vi "VI-Replace Event Type.vi"(7 "Event Data typedef":path, 11 "error in (no error)":errorcluster, 12 "Event Type typedef":path) -> (15 "error out":errorcluster)   [LabVIEW 2015]
uses:
  <vilib>/Utility/traverseref.llb/TRef TravTarget.ctl
  <vilib>/Utility/traverseref.llb/VI Scripting - Traverse.lvlib
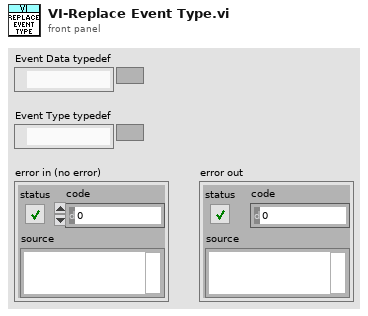
[diagram p1: front panel]
types:
  T1 = typedef "TRef TravTarget.ctl" = enum16{"FP", "BD", "Other"}
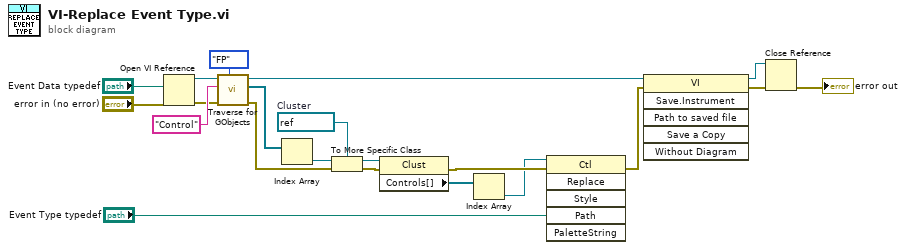
[diagram p0: block diagram]
diagram:
  w7 = refnum<vi> refnum  # Cluster
  n1 = Open VI Reference(vi path="Event Data typedef", error in (no error)="error in (no error)") -> (vi reference=w12:refnum<vi>, error out=w1:errorcluster)  [unwired: 4 in]
  n2 = call <vilib>:"Traverse for GObjects.vi"("Traverse Target"=TRef_TravTarget."FP", "error in (no error)"=w1, "Class Name"="Control", "VI Refnum"=w12) -> ("error out"=w4:errorcluster, "References"=w9:refnum<vi>[], "dup VI Refnum"=w16:refnum<vi>)  [unwired: 4 in, 1 out]
  n3 = Index Array(array=w9) -> (element=w8:refnum<vi>)  [unwired: 1 in]
  n4 = To More Specific Class(target class=w7, reference=w8, error in=w4) -> (specific class reference=w5:refnum<vi>, error out=w6:errorcluster)
  n5 = property class="Clust"(reference=w5, error in=w6) -> (error out=w15:errorcluster, "Controls[]"=w13:refnum<vi>[])  [unwired: 1 out]
  n6 = Index Array(array=w13) -> (element=w14:refnum<vi>)  [unwired: 1 in]
  n7 = invoke class="Ctl" method="Replace"(reference=w14, error in=w15, "Path"="Event Type typedef") -> (error out=w17:errorcluster)  [unwired: 3 in, 5 out]
  n8 = invoke class="VI" method="Save.Instrument"(reference=w16, error in=w17) -> (reference out=w19:refnum<vi>, error out=w18:errorcluster)  [unwired: 4 in, 4 out]
  n9 = Close Reference(reference=w19, error in (no error)=w18) -> (error out=→"error out":errorcluster)
